vi "Command (read) - IP.vi"(7 "timeout ms (100)":i32=100, 8 "error in (no error)":errorcluster, 10 "IP":string, 11 "connection ID in":refnum<k16>) -> (0 "error out":errorcluster, 2 "Position":i32, 3 "connection ID out":refnum<k16>)   [LabVIEW 2016, in "SMD-7615.lvlib" / "eSCL.lvlib"]
doc: "IP - Immediate Position\nRequests present absolute position. This is the calculated trajectory position, which is not always equal to actual position. The position data is assigned a 32-bit value. When sent out in Hexadecimal it will be 8 characters long. When sent out in decimal it will range from 2147483647 to -2147483648."
uses:
  eSCL.lvlib
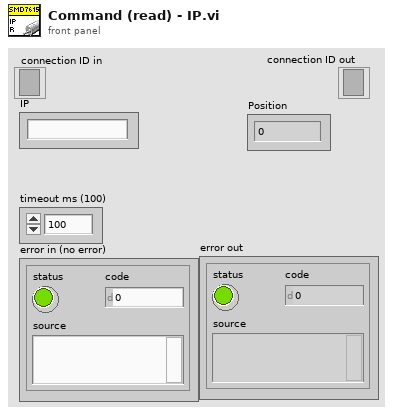
[diagram p1: front panel]
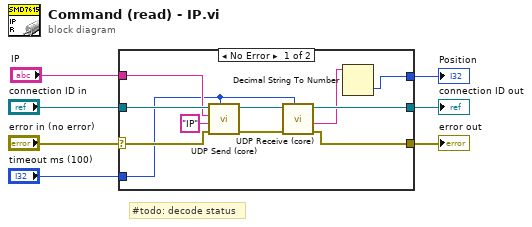
[diagram p0: block diagram]
diagram:
  # "#todo: decode status"
  n1 = case shown="No Error" "error in (no error)" {
    selector: "error in (no error)" -> [w14 w19]
    tunnel: "connection ID in" -> [w13 w20]
    tunnel: [w16 w20] -> w5
    tunnel: [w15 w19] -> w4
    tunnel: "IP" -> [w12 _]
    tunnel: "timeout ms (100)" -> [w10 _]
    tunnel: [w8 _] -> w1
    frame No Error {
      n2 = call "UDP Send (core).vi"("timeout ms (100)"=w10, "error in (no error)"=w14, "Data"="IP", "IP"=w12, "connection ID in"=w13) -> ("error out"=w18:errorcluster, "connection ID out"=w17:refnum<k16>)  [unwired: 5 in]
      n3 = call "UDP Receive (core).vi"("timeout ms (100)"=w10, "error in (no error)"=w18, "connection ID in"=w17) -> ("error out"=w15:errorcluster, "Data"=w9:string, "connection ID out"=w16:refnum<k16>)  [unwired: 4 in, 2 out]
      n4 = Decimal String To Number(string=w9) -> (number=w8:i32)  [unwired: 2 in, 1 out]
    }
    frame Error {
    }
  }
  "connection ID out" <- w5
  "error out" <- w4
  "Position" <- w1
